vi "Configure Common PUSCH Allocation.vi"(0 "VISA resource name":refnum<visa-resource-name>, 1 "Mapping Type (A)":i32(ring) items=["A", "B"], 2 "Start Symbol (0)":i32, 3 "Start RB (0)":i32, 5 "Instance (1)":T3=1, 7 "Carrier Component (1)":T1=1, 9 "Allocation (1)":T2=1, 11 "error in (no error)":errorcluster, 12 "No Symbols (4)":i32=4, 13 "No RBs (1)":i32=1, 14 "Modulation Scheme (Pi/2-BPSK)":i32(ring) items=["Pi/2-BPSK", "QPSK", "16-QAM", "64-QAM", "256-QAM"]) -> (4 "VISA resource name out":refnum<visa-resource-name>, 15 "error out":errorcluster)   [LabVIEW 2015, in "Rohde&Schwarz CMXP NR FR2 Measurement.lvlib"]
doc: "Specifies settings related to the PUSCH allocation, for carrier <no>, allocation <a>.\n\nAttribute:\nRSCMXPNRFR2M_ATTR_COMMON_PUSCH_ALLOCATION\n\nRemote-control command:\nCONFigure:NRMMw:MEAS<i>[:CC<no>]:ALLocation<a>:PUSCh"
uses:
  <instrlib>/Rohde&Schwarz CMXP NR FR2 Measurement/Rohde&Schwarz CMXP NR FR2 Measurement.lvlib
  <instrlib>/Rohde&Schwarz CMXP NR FR2 Measurement/Private/_Instance.ctl
  <instrlib>/Rohde&Schwarz CMXP NR FR2 Measurement/Private/_Allocation.ctl
  <instrlib>/Rohde&Schwarz CMXP NR FR2 Measurement/Private/_Carrier Component.ctl
  <instrlib>/Rohde&Schwarz CMXP NR FR2 Measurement/Private/rsidr_core.llb/rsidr_core.lvlib
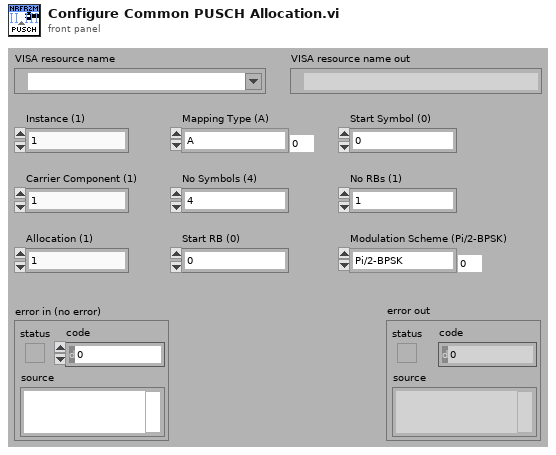
[diagram p1: front panel]
types:
  T1 = typedef "Rohde&Schwarz CMXP NR FR2 Measurement.lvlib/_Carrier Component.ctl" = i32
  T2 = typedef "Rohde&Schwarz CMXP NR FR2 Measurement.lvlib/_Allocation.ctl" = i32
  T3 = typedef "Rohde&Schwarz CMXP NR FR2 Measurement.lvlib/_Instance.ctl" = i32
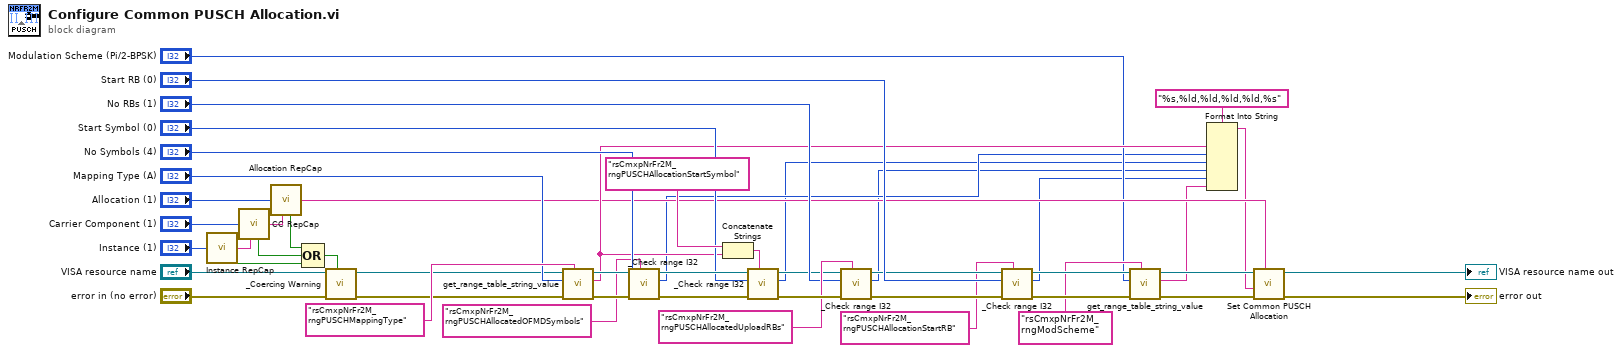
[diagram p0: block diagram]
diagram:
  n1 = call <instrlib>:"Instance RepCap.vi"("Instance In"="Instance (1)") -> ("In Range?"=w44:bool, "RepCap Identifier Out"=w2:string)  [unwired: 1 in]
  n2 = call <instrlib>:"CC RepCap.vi"("CC In"="Carrier Component (1)", "RepCap String In (\"\")"=w2) -> ("In Range?"=w43:bool, "RepCap Identifier Out"=w41:string)
  n3 = call <instrlib>:"Allocation RepCap.vi"("Allocation In"="Allocation (1)", "RepCap String In (\"\")"=w41) -> ("In Range?"=w42:bool, "RepCap Identifier Out"=w15:string)
  n4 = Compound Arithmetic op=OR(w42, w43, w44) -> (w46:bool)
  n5 = call <instrlib>:"_Coercing Warning.vi"("In Range?"=w46, "error in (no error)"="error in (no error)", "VISA resource name"="VISA resource name") -> ("error out"=w38:errorcluster, "VISA resource name out"=w37:refnum<visa-resource-name>)  [unwired: 7 in]
  n6 = call <instrlib>:"get_range_table_string_value.vi"("Range Table ID in"="rsCmxpNrFr2M_rngPUSCHMappingType", "error in"=w38, "I32 input"="Mapping Type (A)", "VISA resource name"=w37) -> ("error out"=w36:errorcluster, "String Value out"=w16:string, "VISA resource name out"=w34:refnum<visa-resource-name>)  [unwired: 5 in]
  n7 = call <instrlib>:"_Check range I32.vi"("Range Table Identifier"="rsCmxpNrFr2M_rngPUSCHAllocatedOFMDSymbols", "error in (no error)"=w36, "I32 Value In"="No Symbols (4)", "VISA resource name"=w34) -> ("error out"=w32:errorcluster, "I32 Value Out"=w8:i32, "VISA resource name out"=w31:refnum<visa-resource-name>)  [unwired: 5 in]
  n8 = Concatenate Strings("rsCmxpNrFr2M_rngPUSCHAllocationStartSymbol", w16) -> (w29:string)
  n9 = call <instrlib>:"_Check range I32.vi"("Range Table Identifier"=w29, "error in (no error)"=w32, "I32 Value In"="Start Symbol (0)", "VISA resource name"=w31) -> ("error out"=w27:errorcluster, "I32 Value Out"=w7:i32, "VISA resource name out"=w24:refnum<visa-resource-name>)  [unwired: 5 in]
  n10 = call <instrlib>:"_Check range I32.vi"("Range Table Identifier"="rsCmxpNrFr2M_rngPUSCHAllocatedUploadRBs", "error in (no error)"=w27, "I32 Value In"="No RBs (1)", "VISA resource name"=w24) -> ("error out"=w23:errorcluster, "I32 Value Out"=w6:i32, "VISA resource name out"=w21:refnum<visa-resource-name>)  [unwired: 5 in]
  n11 = call <instrlib>:"_Check range I32.vi"("Range Table Identifier"="rsCmxpNrFr2M_rngPUSCHAllocationStartRB", "error in (no error)"=w23, "I32 Value In"="Start RB (0)", "VISA resource name"=w21) -> ("error out"=w20:errorcluster, "I32 Value Out"=w5:i32, "VISA resource name out"=w19:refnum<visa-resource-name>)  [unwired: 5 in]
  n12 = call <instrlib>:"get_range_table_string_value.vi"("Range Table ID in"="rsCmxpNrFr2M_rngModScheme", "error in"=w20, "I32 input"="Modulation Scheme (Pi/2-BPSK)", "VISA resource name"=w19) -> ("error out"=w14:errorcluster, "String Value out"=w4:string, "VISA resource name out"=w13:refnum<visa-resource-name>)  [unwired: 5 in]
  n13 = Format Into String(format string="%s,%ld,%ld,%ld,%ld,%s", w16, w8, w7, w6, w5, w4) -> (resulting string=w1:string)  [unwired: 2 in, 1 out]
  n14 = call "Set Common PUSCH Allocation"("Repeated Capabilities"=w15, "error in (no error)"=w14, "Common PUSCH Allocation ()"=w1, "instrument handle"=w13) -> ("error out"=→"error out":errorcluster, "instrument handle out"=→"VISA resource name out":refnum<visa-resource-name>)  [unwired: 6 in]
